vi "Quadratic Roots.vi"() -> ()   [LabVIEW 2019]
panel:
  out "Root 2":dbl
  out "Root 1":dbl
  in  "C":dbl
  in  "B":dbl
  in  "A":dbl
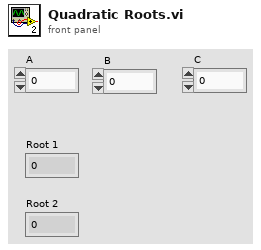
[diagram p1: front panel]
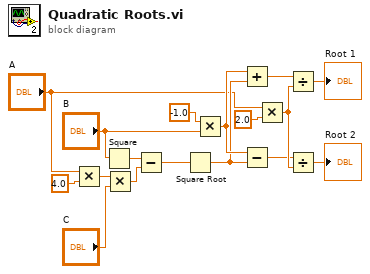
[diagram p0: block diagram]
diagram:
  n1 = Multiply(x="A", y=4.0) -> (x*y=w14:dbl)
  n2 = Square(x="B") -> (x^2=w2:dbl)
  n3 = Multiply(x=w14, y="C") -> (x*y=w3:dbl)
  n4 = Subtract(x=w2, y=w3) -> (x-y=w1:dbl)
  n5 = Square Root(x=w1) -> (sqrt(x)=w11:dbl)
  n6 = Multiply(x=-1.0, y="B") -> (x*y=w12:dbl)
  n7 = Add(x=w12, y=w11) -> (x+y=w8:dbl)
  n8 = Subtract(x=w12, y=w11) -> (x-y=w5:dbl)
  n9 = Multiply(x="A", y=2.0) -> (x*y=w6:dbl)
  n10 = Divide(x=w8, y=w6) -> (x/y=→"Root 1":dbl)
  n11 = Divide(x=w5, y=w6) -> (x/y=→"Root 2":dbl)
